vi "Serialize - JSON.vi"(8 "error in":errorcluster, 11 "PAS Cell Data in":refnum<class "PAS Cell Data.lvclass">) -> (0 "error out":errorcluster, 2 "Serialized JSON":string, 3 "PAS Cell Data out":refnum<class "PAS Cell Data.lvclass">)   [LabVIEW 2014, in "PAS Library.lvlib" / "PAS Cell Data.lvclass"]
uses:
  PAS Cell Data.lvclass
  <vilib>/Analysis/Matrix/Datatypes/RealMatrix.ctl
  PAS Cell Data.lvclass/PAS Cell Data.ctl
  <vilib>/Analysis/Matrix/NI_Matrix.lvlib
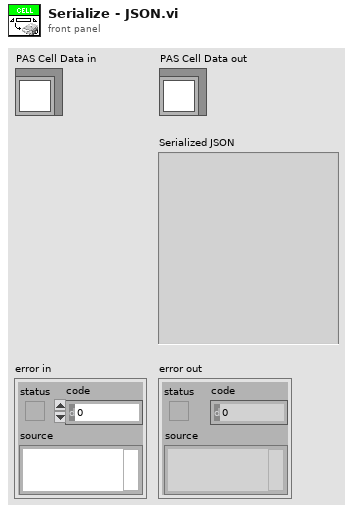
[diagram p1: front panel]
types:
  T1 = typedef "NI_Matrix.lvlib/RealMatrix.ctl" = dbl[][]
  T2 = cluster{"derived":cluster{"f0":sgl, "IA":sgl, "Q":sgl, "max":dbl[], "noiseLim":dbl, "ext":dbl}, "fitData":cluster{"parameters":dbl[], "covariance":T1}, "IABack":dbl, "FittedData":cluster{"Y":sgl[], "dt":dbl}, "MicFreq":cluster{"Y":sgl[], "dt":dbl}, "MicTime":cluster{"Y":i16[], "dt":dbl}, "PhotoDiode":cluster{"Y":i16[], "dt":dbl}, "lRMS":dbl, "phase":cluster{"mic":dbl, "pd":dbl}}
  T3 = cluster{"f0":sgl, "IA":sgl, "Q":sgl, "max":dbl[], "noiseLim":dbl, "abs":dbl}
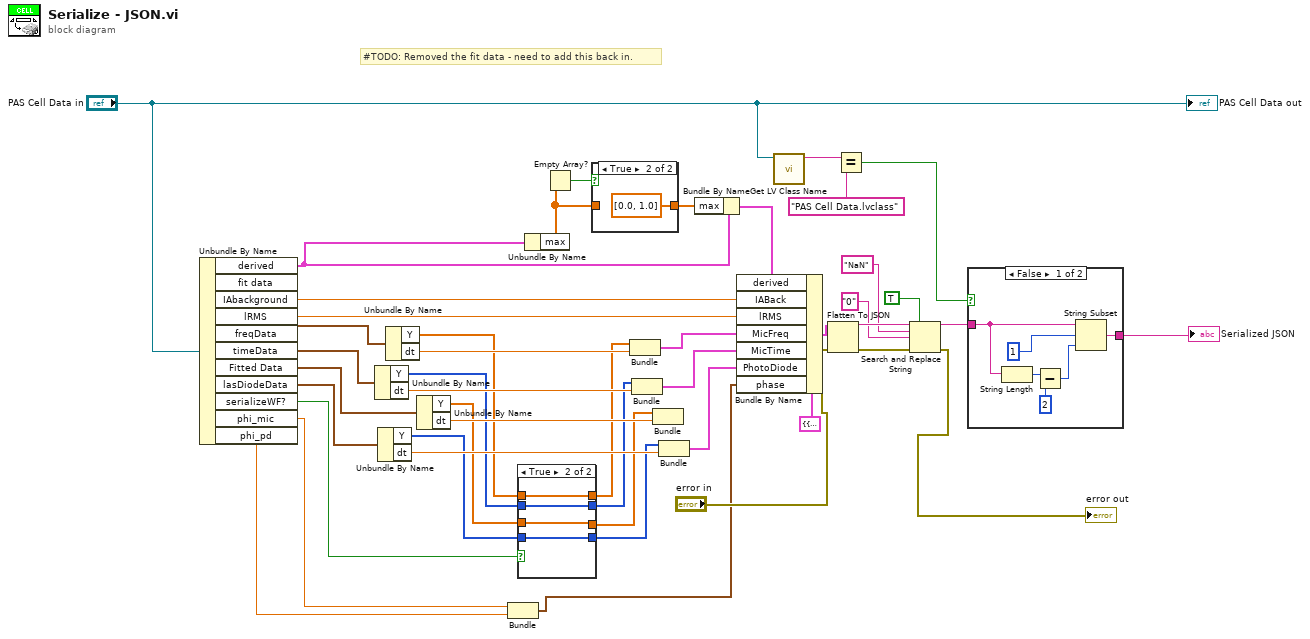
[diagram p0: block diagram]
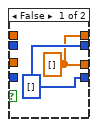
[diagram p2: hidden frame]
diagram:
  # "#TODO: Removed the fit data - need to add this back in."
  n1 = Unbundle By Name("PAS Cell Data in") -> ("derived"=w19:T3, "IAbackground"=w45:dbl, "lRMS"=w44:dbl, "freqData"=w43:waveform(sgl), "timeData"=w39:waveform(i16), "Fitted Data"=w36:waveform(sgl), "lasDiodeData"=w34:waveform(i16), "serializeWF?"=w14:bool, "phi_mic"=w3:dbl, "phi_pd"=w2:dbl)  [unwired: 1 out]
  n2 = Unbundle By Name(w39) -> ("Y"=w8:i16[], "dt"=w40:dbl)
  n3 = Unbundle By Name(w34) -> ("Y"=w6:i16[], "dt"=w35:dbl)
  n4 = Unbundle By Name(w43) -> ("Y"=w9:sgl[], "dt"=w42:dbl)
  n5 = Unbundle By Name(w36) -> ("Y"=w7:sgl[], "dt"=w37:dbl)
  n6 = Bundle("phi_mic"=w3, "phi_pd"=w2) -> (w1:cluster{"phi_mic":dbl, "phi_pd":dbl})  [unwired: 1 in]
  n7 = case shown="True" w14 {
    tunnel: [w47 w48] -> w13
    tunnel: [w47 w50] -> w12
    tunnel: [w46 w51] -> w11
    tunnel: [w46 w49] -> w10
    tunnel: w9 -> [_ w51]
    tunnel: w8 -> [_ w50]
    tunnel: w7 -> [_ w49]
    tunnel: w6 -> [_ w48]
    frame False {
      w47 = i16[] [] ("Y")
      w46 = sgl[] [] ("Y")
    }
    frame True {
    }
  }
  n8 = Unbundle By Name(w19) -> ("max"=w20:dbl[])
  n9 = Empty Array?(array=w20) -> (empty?=w21:bool)
  n10 = case shown="True" w21 {
    tunnel: w20 -> [w52 _]
    tunnel: [w52 dbl[] [0.0, 1.0] ("max")] -> w18
    frame False {
    }
    frame True {
    }
  }
  n11 = Bundle("Y"=w11, "dt"=w42) -> (w41:cluster{"Y":sgl[], "dt":dbl})  [unwired: 1 in]
  n12 = Bundle("Y"=w12, "dt"=w40) -> (w38:cluster{"Y":i16[], "dt":dbl})  [unwired: 1 in]
  n13 = Bundle("Y"=w10, "dt"=w37) -> ()  [unwired: 1 in, 1 out]
  n14 = Bundle("Y"=w13, "dt"=w35) -> (w33:cluster{"Y":i16[], "dt":dbl})  [unwired: 1 in]
  n15 = Bundle By Name(cluster=w19, "max"=w18) -> (w17:T3)
  n16 = Bundle By Name(cluster=T2 {"derived"={"f0"=0.0, "IA"=0.0, "Q"=0.0, "max"=[0.0], "noiseLim"=0.0, "ext"=0.0}, "fitData"={"parameters"=[0.0], "covariance"=[[0.0, 0.0], [0.0, 0.0]]}, "IABack"=0.0, "FittedData"={"Y"=[0.0], "dt"=0.0}, "MicFreq"={"Y"=[0.0], "dt"=0.0}, "MicTime"={"Y"=[0], "dt"=0.0}, "PhotoDiode"={"Y"=[0], "dt"=0.0}, "lRMS"=0.0, "phase"={"mic"=0.0, "pd"=0.0}}, "derived"=w17, "IABack"=w45, "lRMS"=w44, "MicFreq"=w41, "MicTime"=w38, "PhotoDiode"=w33, "phase"=w1) -> (w32:T2)
  n17 = call <vilib>:"Get LV Class Name.vi"("object"="PAS Cell Data in") -> ("class name"=w27:string)  [unwired: 9 in, 1 out]
  n18 = Flatten To JSON(anything=w32, error in (no error)="error in") -> (JSON string=w31:string, 11:w16:errorcluster)  [unwired: 1 in]
  n19 = Equal?(x=w27, y="PAS Cell Data.lvclass") -> (x = y?=w25:bool)
  n20 = Search and Replace String(replace all?=TRUE ("replace all? (F)"), input string=w31, search string="NaN", replace string="0" ("replace string (\"\")"), error in=w16) -> (result string=w24:string, error out=→"error out":errorcluster)  [unwired: 3 in, 2 out]
  n21 = case shown="False" w25 {
    tunnel: w24 -> [w58 w60]
    tunnel: [w54 w60] -> w23
    frame False {
      n22 = String Length(string=w58) -> (length=w57:i32)
      n23 = Subtract(x=w57, y=2) -> (x-y=w55:i32)
      n24 = String Subset(string=w58, offset (0)=1, length (rest)=w55) -> (substring=w54:string)
    }
    frame True {
    }
  }
  "Serialized JSON" <- w23
  "PAS Cell Data out" <- "PAS Cell Data in"
